vi "Run SubVI.vi"(0 "VIリファレンス":refnum<vi>, 1 "VI Window Title":string, 3 "Window Status":T1(ring)=enum."Standard", 5 "Value Ctl Names":string[](array[string]), 9 "Values":variant[](array[variant]), 11 "error in (no error)":errorcluster caption="エラー入力（エラーなし）", 12 "終了まで待機 (F)":bool, 13 "Horizontal alignment":dbl=0.5 min=0.0 max=1.0 step=0.1, 14 "Vertical alignment":dbl=0.5 min=0.0 max=1.0 step=0.1) -> (4 "リファレンス出力":refnum<vi>, 15 "error out":errorcluster caption="エラー出力")   [LabVIEW 2018]
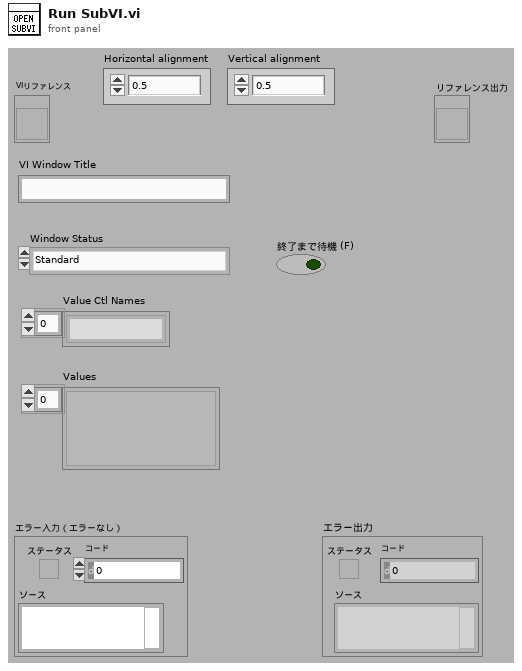
[diagram p1: front panel]
types:
  T1 = enum32{"Invalid", "Standard", "Closed", "Hidden", "Minimized", "Maximized"}
  T2 = enum32{"Bad", "Idle", "Run top level", "Running"}
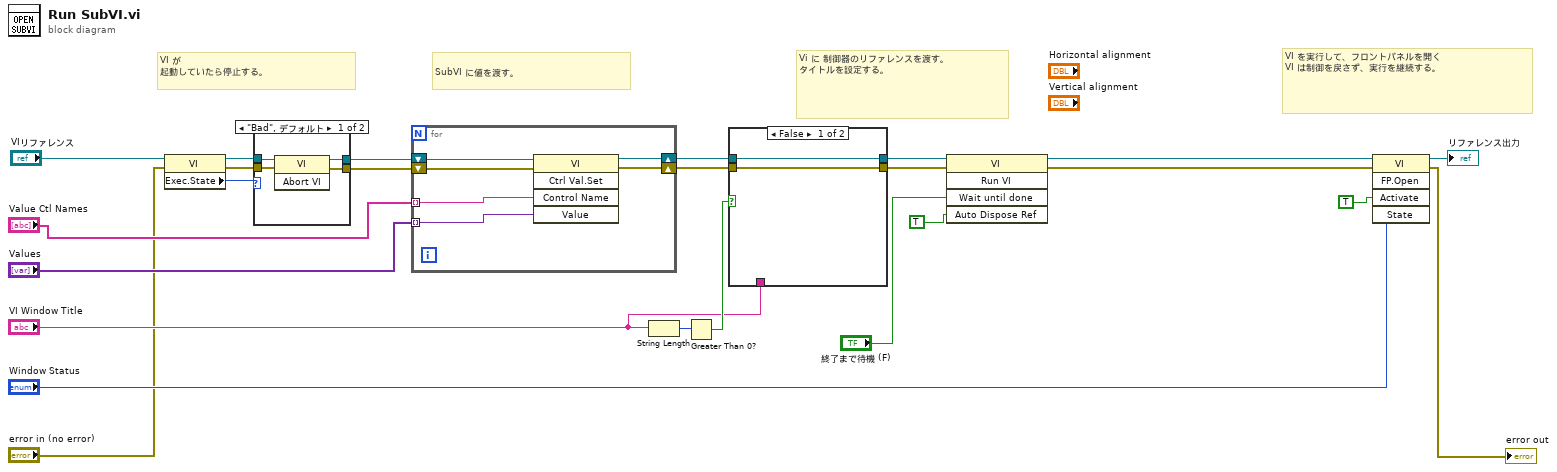
[diagram p0: block diagram]
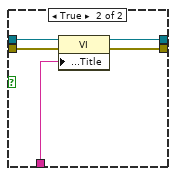
[diagram p2: hidden frame]
diagram:
  # "SubVI に値を渡す。"
  # "VI を実行して、フロントパネルを開く\nVI は制御を戻さず、実行を継続する。"
  # "Vi に 制御器のリファレンスを渡す。\nタイトルを設定する。"
  # "VI が\n起動していたら停止する。"
  n1 = property class="VI"(reference="VIリファレンス", error in="error in (no error)") -> (reference out=w21:refnum<vi>, error out=w22:errorcluster, "Exec.State"=w23:T2)
  n2 = case shown="\"Bad\", デフォルト" w23 {
    tunnel: w22 -> [w28 w29]
    tunnel: w21 -> [w27 w30]
    tunnel: [w26 w30] -> w20
    tunnel: [w25 w29] -> w19
    frame "Bad", Default {
      n3 = invoke class="VI" method="Abort VI"(reference=w27, error in=w28) -> (reference out=w26:refnum<vi>, error out=w25:errorcluster)  [unwired: 1 in, 1 out]
    }
    frame "Idle" {
    }
  }
  n4 = for {
    tunnel: "Value Ctl Names" -> [w31] mode=indexing
    tunnel: "Values" -> [w32] mode=indexing
    shift-right: [w36] -> w16
    shift-left: w20 -> [w35]
    shift-right: [w33] -> w15
    shift-left: w19 -> [w34]
    n5 = invoke class="VI" method="Ctrl Val.Set"(reference=w35, error in=w34, "Control Name"=w31, "Value"=w32) -> (reference out=w36:refnum<vi>, error out=w33:errorcluster)  [unwired: 1 in, 3 out]
  }
  n6 = String Length(string="VI Window Title") -> (length=w9:i32)
  n7 = Greater Than 0?(x=w9) -> (x > 0?=w8:bool)
  n8 = case shown="FALSE" w8 {
    tunnel: w16 -> [w38 w43]
    tunnel: w15 -> [w37 w42]
    tunnel: [w37 w41] -> w12
    tunnel: [w38 w40] -> w11
    tunnel: "VI Window Title" -> [_ w39]
    frame False {
    }
    frame True {
      n9 = property class="VI"(reference=w43, error in=w42, "Front Panel.Title"=w39) -> (reference out=w40:refnum<vi>, error out=w41:errorcluster)
    }
  }
  n10 = invoke class="VI" method="Run VI"(reference=w11, error in=w12, "Wait until done"="終了まで待機 (F)", "Auto Dispose Ref"=TRUE ("リファレンスを自動破棄")) -> (reference out=w2:refnum<vi>, error out=w1:errorcluster)  [unwired: 1 in, 3 out]
  n11 = invoke class="VI" method="FP.Open"(reference=w2, error in=w1, "Activate"=TRUE ("Activate?"), "State"="Window Status") -> (reference out=→"リファレンス出力":refnum<vi>, error out=→"error out":errorcluster)  [unwired: 1 in, 3 out]
